vi "Simplify Method Name.vi"(11 "Method Full Qualified Name":string) -> (3 "Class and Method Only":string)   [LabVIEW 2020, in "Peek Window.lvlib" / "Dynamic Dispatch VI Type.lvclass"]
uses:
  Dynamic Dispatch VI Type.lvclass
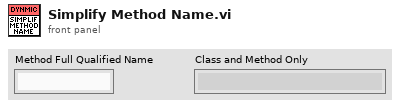
[diagram p1: front panel]
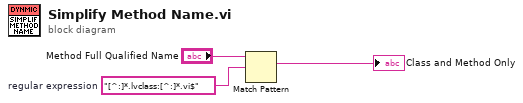
[diagram p0: block diagram]
diagram:
  w2 = "[^:]*.lvclass:[^:]*.vi$"  # regular expression
  n1 = Match Pattern(string="Method Full Qualified Name", regular expression=w2) -> (match substring=→"Class and Method Only":string)  [unwired: 1 in, 3 out]
